vi "Launch Scoring.vi"(11 "Zip":path=path "C:/sol/zip/75.zip") -> (0 "error out":errorcluster, 3 "VI Refnum":refnum<vi>, 5 "App Ref":refnum<vi>)   [LabVIEW 2024, in "Word Search Scorer.lvlib"]
uses:
  Word Search Scorer.lvlib
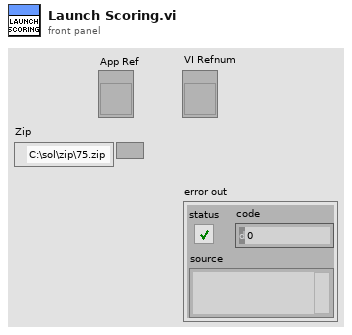
[diagram p1: front panel]
types:
  T1 = enum32{"invalid app kind", "Development System", "Run Time System", "Student Edition", "Embedded LabVIEW", "Evaluation", "Custom"}
  T2 = enum32{"Invalid", "Standard", "Closed", "Hidden", "Minimized", "Maximized"}
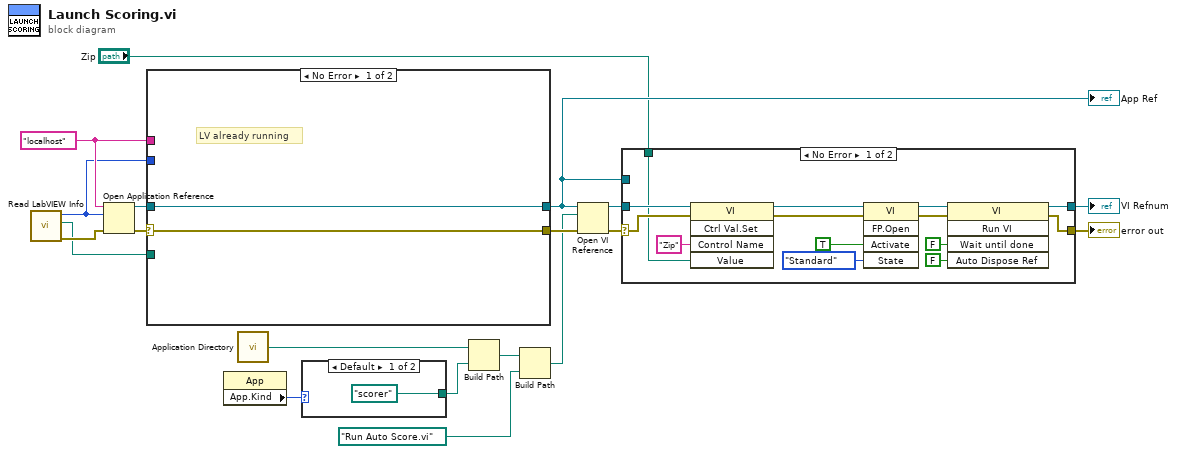
[diagram p0: block diagram]
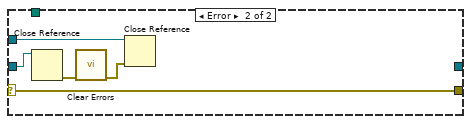
[diagram p2: hidden frame]
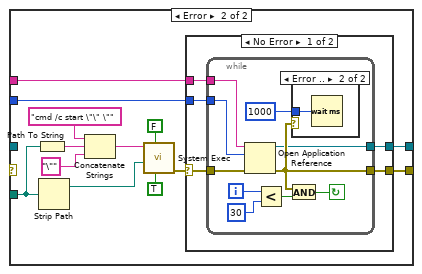
[diagram p3: hidden frame]
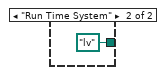
[diagram p6: hidden frame]
diagram:
  w16 = "localhost" ("machine name (\"\":  open local reference)")
  n1 = call "Read LabVIEW Info.vi"() -> ("error out"=w2:errorcluster, "LabVIEW Path"=w1:path, "VI Server Port"=w3:u16)  [unwired: 9 in]
  n2 = Open Application Reference(8:w2, 10:w3, 11:w16) -> (0:w18:errorcluster, 3:w17:refnum<vi>)  [unwired: 1 in]
  n3 = case shown="No Error" w18 {
    selector: w18 -> [w21 _]
    tunnel: [w21 w26] -> w19
    tunnel: w1 -> [_ w34]
    tunnel: w17 -> [w20 _]
    tunnel: w3 -> [_ w28]
    tunnel: [w20 w27] -> w7
    tunnel: w16 -> [_ w25]
    frame No Error {
      # "LV already running"
    }
    frame Error {
      n4 = Path To String(path=w34) -> (string=w32:string)
      n5 = Strip Path(path=w34) -> (stripped path=w31:path)  [unwired: 1 out]
      n6 = Concatenate Strings("cmd /c start \"\" \"", w32, "\"" ("string")) -> (w30:string)
      n7 = call <vilib>:"System Exec.vi"("run minimized? (F)"=TRUE, "wait until completion? (T)"=FALSE, "working directory"=w31, "command line"=w30) -> ("error out"=w29:errorcluster)  [unwired: 4 in, 3 out]
      n8 = case shown="No Error" w29 {
        selector: w29 -> [w39 w51]
        tunnel: w28 -> [w38 _]
        tunnel: [w37 _] -> w27
        tunnel: [w36 w51] -> w26
        tunnel: w25 -> [w35 _]
        frame No Error {
          n9 = while {
            tunnel: w38 -> [w47]
            tunnel: [w46] -> w37
            tunnel: w35 -> [w45]
            tunnel: w39 -> [w48]
            tunnel: [w49] -> w36
            i -> [w44]
            stop <- w41 continue-if-true
            n10 = Open Application Reference(8:w48, 10:w47, 11:w45) -> (0:w49:errorcluster, 3:w46:refnum<vi>)  [unwired: 1 in]
            n11 = Less?(x=w44, y=30) -> (x < y?=w42:bool)
            n12 = And(x=w49, y=w42) -> (x .and. y?=w41:bool)
            n13 = case shown="Error .." w49 {
              tunnel: u32 1000 ("milliseconds to wait") -> [_ w50]
              frame No Error {
              }
              frame Error {
                n14 = Wait (ms)(milliseconds to wait=w50) -> ()  [unwired: 1 out]
              }
            }
          }
        }
        frame Error {
        }
      }
    }
  }
  "App Ref" <- w7
  n15 = property class="App"() -> ("App.Kind"=w14:T1)  [unwired: 2 in, 2 out]
  n16 = call <vilib>:"Application Directory.vi"() -> ("Application Directory"=w13:path)
  n17 = case shown="Default" w14 {
    tunnel: [path "scorer" ("name or relative path") path "lv" ("name or relative path")] -> w11
    frame Default {
    }
    frame "Run Time System" {
    }
  }
  n18 = Build Path(base path=w13, name or relative path=w11) -> (appended path=w12:path)
  n19 = Build Path(base path=w12, name or relative path=path "Run Auto Score.vi") -> (appended path=w10:path)
  n20 = Open VI Reference(application reference (local)=w7, vi path=w10, error in (no error)=w19) -> (vi reference=w8:refnum<vi>, error out=w9:errorcluster)  [unwired: 3 in]
  n21 = case shown="No Error" w9 {
    selector: w9 -> [w67 w68]
    tunnel: w8 -> [w66 w72]
    tunnel: w7 -> [_ w71]
    tunnel: [w61 w68] -> w5
    tunnel: "Zip" -> [w64 _]
    tunnel: [w60 _] -> w4
    frame No Error {
      n22 = invoke class="VI" method="Ctrl Val.Set"(reference=w66, error in=w67, "Control Name"="Zip", "Value"=w64) -> (reference out=w59:refnum<vi>, error out=w58:errorcluster)  [unwired: 1 in, 3 out]
      n23 = invoke class="VI" method="FP.Open"(reference=w59, error in=w58, "Activate"=TRUE ("Activate?"), "State"=T2."Standard") -> (reference out=w57:refnum<vi>, error out=w56:errorcluster)  [unwired: 1 in, 3 out]
      n24 = invoke class="VI" method="Run VI"(reference=w57, error in=w56, "Wait until done"=FALSE ("Wait Until Done"), "Auto Dispose Ref"=FALSE ("Auto Dispose Reference")) -> (reference out=w60:refnum<vi>, error out=w61:errorcluster)  [unwired: 1 in, 3 out]
    }
    frame Error {
      n25 = Close Reference(reference=w72) -> (error out=w70:errorcluster)  [unwired: 1 in]
      n26 = call <vilib>:"Clear Errors.vi"("error in (no error)"=w70) -> ("error out"=w69:errorcluster)  [unwired: 5 in, 1 out]
      n27 = Close Reference(reference=w71, error in (no error)=w69) -> ()  [unwired: 1 out]
    }
  }
  "error out" <- w5
  "VI Refnum" <- w4
